vi "vi.under.test.vi"(10 "B":i32, 11 "A":i32) -> (3 "SUM":i32)   [LabVIEW 2020]
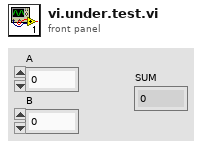
[diagram p1: front panel]
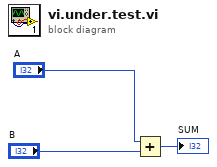
[diagram p0: block diagram]
diagram:
  n1 = Add(x="A", y="B") -> (x+y=→"SUM":i32)
